vi "Test serial serialization.vi"() -> ()   [LabVIEW 2014]
uses:
  <userlib>/Serialization/JSON Serializer/JSON Serializer.lvclass
  Reusable/CRDS/Main/CRDS.lvclass
  Reusable/CRDS/Cell/CRDS Cell.lvclass
  reusable/Switch/Switch.lvclass
  Reusable/CRDS/Cell/Get Tau Method.ctl
  <userlib>/Serialization/JSON Deserializer/JSON Deserializer.lvclass
  Alicat/AlicatCommBank/AlicatCommBank.lvclass
  Alicat/Alicat Controller/Alicat Controller.lvclass
  Alicat/Alicat.lvclass
  Alicat/Controls/Gas.ctl
panel:
  in  "Path Embedding":T1(ring)
  in  "Include default value fields?":bool=TRUE
  out "String":string
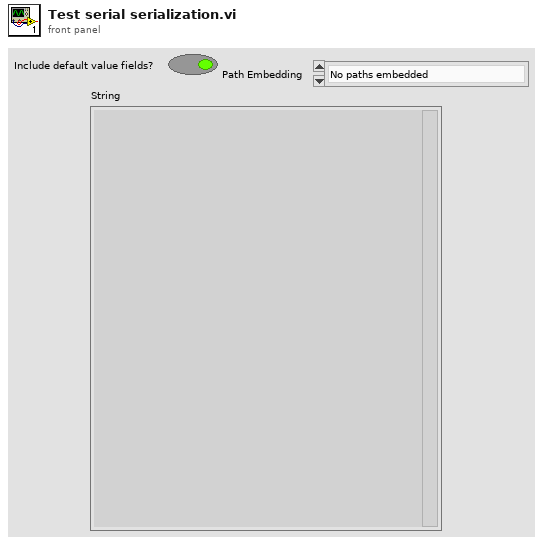
[diagram p1: front panel]
types:
  T1 = enum16{"No paths embedded", "One path with each object", "All paths with top object"}
  T2 = typedef "Alicat.lvlib/Alicat.lvclass/Gas.ctl" = enum16{"Air", "Ar", "CH4", "CO", "CO2", "C2H6", "H2", "He", "N2", "NO", "Ne", "O2", "C3H8", "n-C4H10", "C2H2", "C2H4", "i-C2H10", "Kr", "Xe"}
  T3 = typedef "Base CRDS Lib.lvlib/Get Tau Method.ctl" = enum8{"DFT-1", "DFT-5", "LRS"}
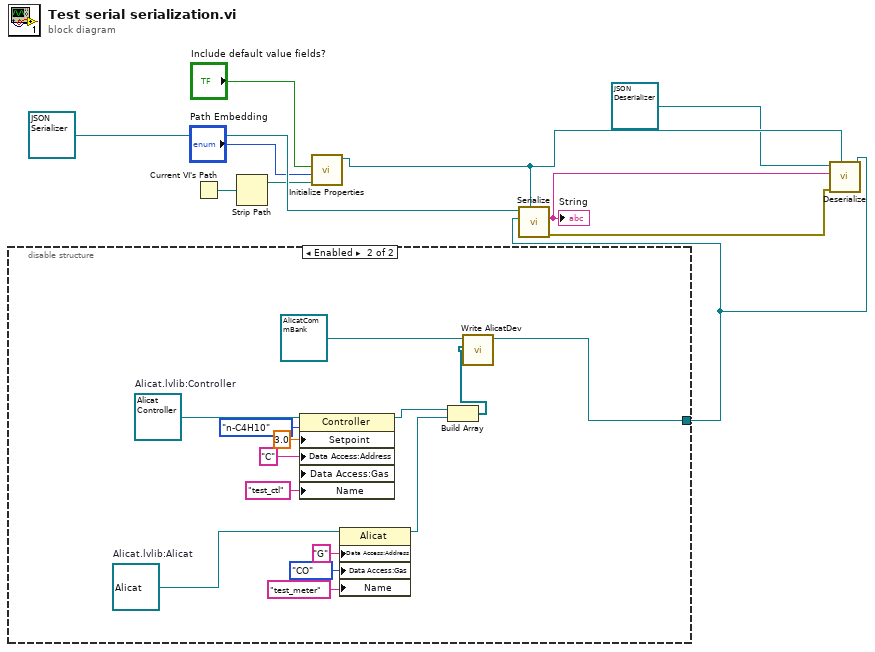
[diagram p0: block diagram]
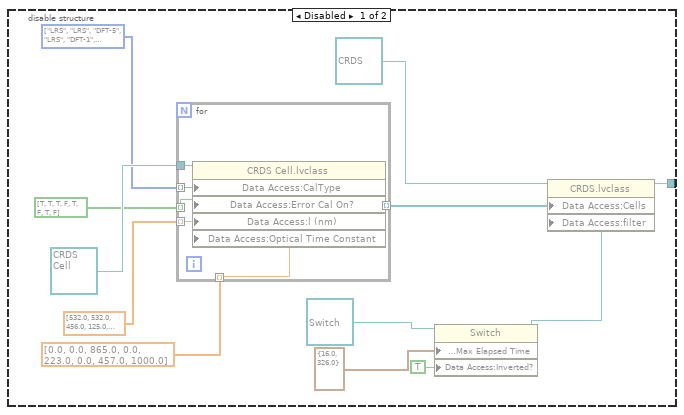
[diagram p2: hidden frame]
diagram:
  n1 = disable-structure shown="Enabled" {
    disable-tunnel: [w12 w41] -> w1
    frame Disabled {
      w19 = T3[] [enum."LRS", enum."LRS", enum."DFT-5", enum."LRS", enum."DFT-1", enum."DFT-5", enum."LRS", enum."DFT-5"] items=["DFT-1", "DFT-5", "LRS"]
      n2 = for {
        tunnel: refnum<class "CRDS Cell.lvclass"> refnum ("Base CRDS Lib.lvlib:CRDS Cell") -> [w28]
        tunnel: [w27] -> w20 mode=indexing
        tunnel: w19 -> [w26] mode=indexing
        tunnel: bool[] [TRUE, TRUE, TRUE, FALSE, TRUE, FALSE, TRUE, FALSE] -> [w25] mode=indexing
        tunnel: sgl[] [532.0, 532.0, 456.0, 125.0, 532.0, 332.0, 532.0, 667.0] -> [w24] mode=indexing
        tunnel: sgl[] [0.0, 0.0, 865.0, 0.0, 223.0, 0.0, 457.0, 1000.0] -> [w23] mode=indexing
        n3 = property class="CRDS Cell.lvclass"(reference=w28, "Data Access:CalType"=w26, "Data Access:Error Cal On?"=w25, "Data Access:l (nm)"=w24, "Data Access:Optical Time Constant"=w23) -> (reference out=w27:refnum<class "CRDS Cell.lvclass">)  [unwired: 1 in, 1 out]
      }
      n4 = property class="Switch"(reference=refnum<class "Switch.lvclass"> refnum ("filter"), "Data Access:Max Elapsed Time"=cluster{"true":dbl, "false":dbl} {"true"=16.0, "false"=326.0} ("Max Elapsed Time"), "Data Access:Inverted?"=TRUE ("Inverted?")) -> (reference out=w13:refnum<class "Switch.lvclass">)  [unwired: 1 in, 1 out]
      n5 = property class="CRDS.lvclass"(reference=refnum<class "CRDS.lvclass"> refnum ("Base CRDS Lib.lvlib:CRDS.lvclass"), "Data Access:Cells"=w20, "Data Access:filter"=w13) -> (reference out=w12:refnum<class "CRDS.lvclass">)  [unwired: 1 in, 1 out]
    }
    frame Enabled {
      w39 = refnum<class "Alicat.lvclass"> refnum  # Alicat.lvlib:Alicat
      w40 = refnum<class "Alicat Controller.lvclass"> refnum  # Alicat.lvlib:Controller
      n6 = property class="Controller"(reference=w40, "Setpoint"=sgl 3.0, "Data Access:Address"="C" ("Address"), "Data Access:Gas"=Gas."n-C4H10" ("Gas"), "Name"="test_ctl") -> (reference out=w30:refnum<class "Alicat Controller.lvclass">)  [unwired: 1 in, 1 out]
      n7 = property class="Alicat"(reference=w39, "Data Access:Address"="G" ("Address"), "Data Access:Gas"=Gas."CO" ("Gas"), "Name"="test_meter") -> (reference out=w31:refnum<class "Alicat.lvclass">)  [unwired: 1 in, 1 out]
      n8 = Build Array(w30, w31) -> (w29:refnum<class "Alicat.lvclass">[])
      n9 = call "Write AlicatDev.vi"("AlicatDev"=w29, "AlicatCommBank in"=refnum<class "AlicatCommBank.lvclass"> refnum ("Alicat.lvlib:AC Comm")) -> ("AlicatCommBank out"=w41:refnum<class "AlicatCommBank.lvclass">)  [unwired: 8 in, 1 out]
    }
  }
  n10 = Current VI's Path() -> (path=w7:path)
  n11 = Strip Path(path=w7) -> (stripped path=w6:path)  [unwired: 1 out]
  n12 = call <userlib>:"Initialize Properties.vi"("Absolute Path For Dynamic Loading"=w6, "Path Embedding"="Path Embedding", "Include all fields?"="Include default value fields?") -> ("Formatter out"=w5:refnum<class "Formatter.lvclass">)  [unwired: 8 in]
  n13 = call <userlib>:"Serialize.vi"("Formatter (defaults)"=w5, "Serializable"=w1, "Serializer"=refnum<class "JSON Serializer.lvclass"> refnum ("JSON Serializer.lvclass")) -> ("error out"=w2:errorcluster, "String"=w3:string)  [unwired: 6 in, 1 out]
  "String" <- w3
  n14 = call <userlib>:"Deserialize.vi"("Target Type (Serializable.lvclass)"=w1, "Formatter (defaults)"=w5, "error in (no error)"=w2, "String"=w3, "Deserializer"=refnum<class "JSON Deserializer.lvclass"> refnum ("JSON Deserializer.lvclass")) -> ()  [unwired: 4 in, 3 out]
